vi "MH_WriteTestPTUFileV2.vi"(8 "entrée d'erreur":errorcluster) -> (0 "sortie d'erreur":errorcluster, 3 "refnum Out":refnum<file>)   [LabVIEW 2019]
panel:
  out "Value":u32[](array[numeric])
  out "Records":u32[](array[numeric])
  in  "Path":path
  in  "TagArray":T1(array[cluster])=[{"TagIdent"="File_GUID", "TagIndex"=-1, "TagType"=1073872895, "TagValue"=40, "TagAuxData"="{197B8EE0-02FE-45EA-A6B5-3F8BBDE2D882}\u0000\u0000"}, {"TagIdent"="File_AssuredContent", "TagIndex"=-1, "TagType"=1073872895, "TagValue"=32, "TagAuxData"="MultiHarp: HWSETG SWSETG\u0000\u0000\u0000\u0000\u0000\u0000\u0000\u0000"}, {"TagIdent"="CreatorSW_ContentVersion", "TagIndex"=-1, "TagType"=1073872895, "TagValue"=8, "TagAuxData"="1.0\u0000\u0000\u0000\u0000\u0000"}, {"TagIdent"="CreatorSW_Name", "TagIndex"=-1, "TagType"=1073872895, "TagValue"=16, "TagAuxData"="MultiHarp AcqUI\u0000"}, {"TagIdent"="CreatorSW_Version", "TagIndex"=-1, "TagType"=1073872895, "TagValue"=8, "TagAuxData"="3.0.0.0\u0000"}, {"TagIdent"="File_CreatingTime", "TagIndex"=-1, "TagType"=553648136, "TagValue"=4676398420989345414, "TagAuxData"=""}, {"TagIdent"="File_Comment", "TagIndex"=-1, "TagType"=1073872895, "TagValue"=8, "TagAuxData"="T2 Mode\u0000"}, {"TagIdent"="Measurement_Mode", "TagIndex"=-1, "TagType"=268435464, "TagValue"=2, "TagAuxData"=""}, {"TagIdent"="Measurement_SubMode", "TagIndex"=-1, "TagType"=268435464, "TagValue"=0, "TagAuxData"=""}, {"TagIdent"="TTResult_StopReason", "TagIndex"=-1, "TagType"=268435464, "TagValue"=0, "TagAuxData"=""}, {"TagIdent"="Fast_Load_End", "TagIndex"=-1, "TagType"=-65528, "TagValue"=0, "TagAuxData"=""}, {"TagIdent"="TTResultFormat_TTTRRecType", "TagIndex"=-1, "TagType"=268435464, "TagValue"=66055, "TagAuxData"=""}, {"TagIdent"="TTResultFormat_BitsPerRecord", "TagIndex"=-1, "TagType"=268435464, "TagValue"=32, "TagAuxData"=""}, {"TagIdent"="MeasDesc_BinningFactor", "TagIndex"=-1, "TagType"=268435464, "TagValue"=32, "TagAuxData"=""}, {"TagIdent"="MeasDesc_Offset", "TagIndex"=-1, "TagType"=268435464, "TagValue"=0, "TagAuxData"=""}, {"TagIdent"="MeasDesc_AcquisitionTime", "TagIndex"=-1, "TagType"=268435464, "TagValue"=900000, "TagAuxData"=""}, {"TagIdent"="MeasDesc_StopAt", "TagIndex"=-1, "TagType"=268435464, "TagValue"=4294967295, "TagAuxData"=""}, {"TagIdent"="MeasDesc_StopOnOvfl", "TagIndex"=-1, "TagType"=8, "TagValue"=0, "TagAuxData"=""}, {"TagIdent"="MeasDesc_Restart", "TagIndex"=-1, "TagType"=8, "TagValue"=0, "TagAuxData"=""}, {"TagIdent"="CurSWSetting_DispLog", "TagIndex"=-1, "TagType"=8, "TagValue"=-1, "TagAuxData"=""}, {"TagIdent"="CurSWSetting_DispAxisTimeFrom", "TagIndex"=-1, "TagType"=268435464, "TagValue"=1, "TagAuxData"=""}, {"TagIdent"="CurSWSetting_DispAxisTimeTo", "TagIndex"=-1, "TagType"=268435464, "TagValue"=120, "TagAuxData"=""}, {"TagIdent"="CurSWSetting_DispAxisCountFrom", "TagIndex"=-1, "TagType"=268435464, "TagValue"=1, "TagAuxData"=""}, {"TagIdent"="CurSWSetting_DispAxisCountTo", "TagIndex"=-1, "TagType"=268435464, "TagValue"=10000, "TagAuxData"=""}, {"TagIdent"="CurSWSetting_DispCurves", "TagIndex"=-1, "TagType"=268435464, "TagValue"=16, "TagAuxData"=""}, {"TagIdent"="CurSWSetting_DispCurve_MapTo", "TagIndex"=0, "TagType"=268435464, "TagValue"=0, "TagAuxData"=""}, {"TagIdent"="CurSWSetting_DispCurve_Show", "TagIndex"=0, "TagType"=8, "TagValue"=-1, "TagAuxData"=""}, {"TagIdent"="CurSWSetting_DispCurve_MapTo", "TagIndex"=1, "TagType"=268435464, "TagValue"=1, "TagAuxData"=""}, {"TagIdent"="CurSWSetting_DispCurve_Show", "TagIndex"=1, "TagType"=8, "TagValue"=-1, "TagAuxData"=""}, {"TagIdent"="CurSWSetting_DispCurve_MapTo", "TagIndex"=2, "TagType"=268435464, "TagValue"=2, "TagAuxData"=""}, {"TagIdent"="CurSWSetting_DispCurve_Show", "TagIndex"=2, "TagType"=8, "TagValue"=-1, "TagAuxData"=""}, {"TagIdent"="CurSWSetting_DispCurve_MapTo", "TagIndex"=3, "TagType"=268435464, "TagValue"=3, "TagAuxData"=""}, {"TagIdent"="CurSWSetting_DispCurve_Show", "TagIndex"=3, "TagType"=8, "TagValue"=-1, "TagAuxData"=""}, {"TagIdent"="CurSWSetting_DispCurve_MapTo", "TagIndex"=4, "TagType"=268435464, "TagValue"=4, "TagAuxData"=""}, {"TagIdent"="CurSWSetting_DispCurve_Show", "TagIndex"=4, "TagType"=8, "TagValue"=-1, "TagAuxData"=""}, {"TagIdent"="CurSWSetting_DispCurve_MapTo", "TagIndex"=5, "TagType"=268435464, "TagValue"=5, "TagAuxData"=""}, {"TagIdent"="CurSWSetting_DispCurve_Show", "TagIndex"=5, "TagType"=8, "TagValue"=-1, "TagAuxData"=""}, {"TagIdent"="CurSWSetting_DispCurve_MapTo", "TagIndex"=6, "TagType"=268435464, "TagValue"=6, "TagAuxData"=""}, {"TagIdent"="CurSWSetting_DispCurve_Show", "TagIndex"=6, "TagType"=8, "TagValue"=-1, "TagAuxData"=""}, {"TagIdent"="CurSWSetting_DispCurve_MapTo", "TagIndex"=7, "TagType"=268435464, "TagValue"=7, "TagAuxData"=""}, {"TagIdent"="CurSWSetting_DispCurve_Show", "TagIndex"=7, "TagType"=8, "TagValue"=-1, "TagAuxData"=""}, {"TagIdent"="CurSWSetting_DispCurve_MapTo", "TagIndex"=8, "TagType"=268435464, "TagValue"=8, "TagAuxData"=""}, {"TagIdent"="CurSWSetting_DispCurve_Show", "TagIndex"=8, "TagType"=8, "TagValue"=-1, "TagAuxData"=""}, {"TagIdent"="CurSWSetting_DispCurve_MapTo", "TagIndex"=9, "TagType"=268435464, "TagValue"=9, "TagAuxData"=""}, {"TagIdent"="CurSWSetting_DispCurve_Show", "TagIndex"=9, "TagType"=8, "TagValue"=-1, "TagAuxData"=""}, {"TagIdent"="CurSWSetting_DispCurve_MapTo", "TagIndex"=10, "TagType"=268435464, "TagValue"=10, "TagAuxData"=""}, {"TagIdent"="CurSWSetting_DispCurve_Show", "TagIndex"=10, "TagType"=8, "TagValue"=-1, "TagAuxData"=""}, {"TagIdent"="CurSWSetting_DispCurve_MapTo", "TagIndex"=11, "TagType"=268435464, "TagValue"=11, "TagAuxData"=""}, {"TagIdent"="CurSWSetting_DispCurve_Show", "TagIndex"=11, "TagType"=8, "TagValue"=-1, "TagAuxData"=""}, {"TagIdent"="CurSWSetting_DispCurve_MapTo", "TagIndex"=12, "TagType"=268435464, "TagValue"=12, "TagAuxData"=""}, {"TagIdent"="CurSWSetting_DispCurve_Show", "TagIndex"=12, "TagType"=8, "TagValue"=-1, "TagAuxData"=""}, {"TagIdent"="CurSWSetting_DispCurve_MapTo", "TagIndex"=13, "TagType"=268435464, "TagValue"=13, "TagAuxData"=""}, {"TagIdent"="CurSWSetting_DispCurve_Show", "TagIndex"=13, "TagType"=8, "TagValue"=-1, "TagAuxData"=""}, {"TagIdent"="CurSWSetting_DispCurve_MapTo", "TagIndex"=14, "TagType"=268435464, "TagValue"=14, "TagAuxData"=""}, {"TagIdent"="CurSWSetting_DispCurve_Show", "TagIndex"=14, "TagType"=8, "TagValue"=-1, "TagAuxData"=""}, {"TagIdent"="CurSWSetting_DispCurve_MapTo", "TagIndex"=15, "TagType"=268435464, "TagValue"=15, "TagAuxData"=""}, {"TagIdent"="CurSWSetting_DispCurve_Show", "TagIndex"=15, "TagType"=8, "TagValue"=-1, "TagAuxData"=""}, {"TagIdent"="HW_Type", "TagIndex"=-1, "TagType"=1073872895, "TagValue"=24, "TagAuxData"="MultiHarp 150 4P\u0000\u0000\u0000\u0000\u0000\u0000\u0000\u0000"}, {"TagIdent"="HW_PartNo", "TagIndex"=-1, "TagType"=1073872895, "TagValue"=8, "TagAuxData"="930043\u0000\u0000"}, {"TagIdent"="HW_Version", "TagIndex"=-1, "TagType"=1073872895, "TagValue"=8, "TagAuxData"="1.0\u0000\u0000\u0000\u0000\u0000"}, {"TagIdent"="HW_SerialNo", "TagIndex"=-1, "TagType"=1073872895, "TagValue"=8, "TagAuxData"="1043897\u0000"}, {"TagIdent"="HW_Features", "TagIndex"=-1, "TagType"=285212680, "TagValue"=183, "TagAuxData"=""}, {"TagIdent"="HW_BaseResolution", "TagIndex"=-1, "TagType"=536870920, "TagValue"=4437731733528994965, "TagAuxData"=""}, {"TagIdent"="HW_InpChannels", "TagIndex"=-1, "TagType"=268435464, "TagValue"=4, "TagAuxData"=""}, {"TagIdent"="HW_ExternalRefClock", "TagIndex"=-1, "TagType"=8, "TagValue"=0, "TagAuxData"=""}, {"TagIdent"="HW_ExternalDevices", "TagIndex"=-1, "TagType"=268435464, "TagValue"=0, "TagAuxData"=""}, {"TagIdent"="HWTriggerOut_Period", "TagIndex"=-1, "TagType"=536870920, "TagValue"=4502148214488346441, "TagAuxData"=""}, {"TagIdent"="HWTriggerOut_On", "TagIndex"=-1, "TagType"=8, "TagValue"=0, "TagAuxData"=""}, {"TagIdent"="HW_InputHysteresis", "TagIndex"=-1, "TagType"=8, "TagValue"=0, "TagAuxData"=""}, {"TagIdent"="HWSync_Divider", "TagIndex"=-1, "TagType"=268435464, "TagValue"=1, "TagAuxData"=""}, {"TagIdent"="HWSync_TrgLevel", "TagIndex"=-1, "TagType"=268435464, "TagValue"=-10, "TagAuxData"=""}, {"TagIdent"="HWSync_TrgEdge", "TagIndex"=-1, "TagType"=268435464, "TagValue"=0, "TagAuxData"=""}, {"TagIdent"="HWSync_Offset", "TagIndex"=-1, "TagType"=268435464, "TagValue"=27000, "TagAuxData"=""}, {"TagIdent"="HWSync_TdCode", "TagIndex"=-1, "TagType"=268435464, "TagValue"=0, "TagAuxData"=""}, {"TagIdent"="HWInpChan_TrgLevel", "TagIndex"=0, "TagType"=268435464, "TagValue"=-150, "TagAuxData"=""}, {"TagIdent"="HWInpChan_TrgEdge", "TagIndex"=0, "TagType"=268435464, "TagValue"=0, "TagAuxData"=""}, {"TagIdent"="HWInpChan_Offset", "TagIndex"=0, "TagType"=268435464, "TagValue"=0, "TagAuxData"=""}, {"TagIdent"="HWInpChan_Enabled", "TagIndex"=0, "TagType"=8, "TagValue"=-1, "TagAuxData"=""}, {"TagIdent"="HWInpChan_TdCode", "TagIndex"=0, "TagType"=268435464, "TagValue"=0, "TagAuxData"=""}, {"TagIdent"="HWInpChan_TrgLevel", "TagIndex"=1, "TagType"=268435464, "TagValue"=-150, "TagAuxData"=""}, {"TagIdent"="HWInpChan_TrgEdge", "TagIndex"=1, "TagType"=268435464, "TagValue"=0, "TagAuxData"=""}, {"TagIdent"="HWInpChan_Offset", "TagIndex"=1, "TagType"=268435464, "TagValue"=0, "TagAuxData"=""}, {"TagIdent"="HWInpChan_Enabled", "TagIndex"=1, "TagType"=8, "TagValue"=-1, "TagAuxData"=""}, {"TagIdent"="HWInpChan_TdCode", "TagIndex"=1, "TagType"=268435464, "TagValue"=0, "TagAuxData"=""}, {"TagIdent"="HWInpChan_TrgLevel", "TagIndex"=2, "TagType"=268435464, "TagValue"=-50, "TagAuxData"=""}, {"TagIdent"="HWInpChan_TrgEdge", "TagIndex"=2, "TagType"=268435464, "TagValue"=0, "TagAuxData"=""}, {"TagIdent"="HWInpChan_Offset", "TagIndex"=2, "TagType"=268435464, "TagValue"=0, "TagAuxData"=""}, {"TagIdent"="HWInpChan_Enabled", "TagIndex"=2, "TagType"=8, "TagValue"=-1, "TagAuxData"=""}, {"TagIdent"="HWInpChan_TdCode", "TagIndex"=2, "TagType"=268435464, "TagValue"=0, "TagAuxData"=""}, {"TagIdent"="HWInpChan_TrgLevel", "TagIndex"=3, "TagType"=268435464, "TagValue"=-50, "TagAuxData"=""}, {"TagIdent"="HWInpChan_TrgEdge", "TagIndex"=3, "TagType"=268435464, "TagValue"=0, "TagAuxData"=""}, {"TagIdent"="HWInpChan_Offset", "TagIndex"=3, "TagType"=268435464, "TagValue"=0, "TagAuxData"=""}, {"TagIdent"="HWInpChan_Enabled", "TagIndex"=3, "TagType"=8, "TagValue"=-1, "TagAuxData"=""}, {"TagIdent"="HWInpChan_TdCode", "TagIndex"=3, "TagType"=268435464, "TagValue"=0, "TagAuxData"=""}, {"TagIdent"="MeasDesc_Resolution", "TagIndex"=-1, "TagType"=536870920, "TagValue"=4437731733528994965, "TagAuxData"=""}, {"TagIdent"="HW_Markers", "TagIndex"=-1, "TagType"=268435464, "TagValue"=4, "TagAuxData"=""}, {"TagIdent"="HWMarkers_RisingEdge", "TagIndex"=0, "TagType"=8, "TagValue"=0, "TagAuxData"=""}, {"TagIdent"="HWMarkers_RisingEdge", "TagIndex"=1, "TagType"=8, "TagValue"=0, "TagAuxData"=""}, {"TagIdent"="HWMarkers_RisingEdge", "TagIndex"=2, "TagType"=8, "TagValue"=0, "TagAuxData"=""}, {"TagIdent"="HWMarkers_RisingEdge", "TagIndex"=3, "TagType"=8, "TagValue"=0, "TagAuxData"=""}, {"TagIdent"="HWMarkers_Enabled", "TagIndex"=0, "TagType"=8, "TagValue"=-1, "TagAuxData"=""}, {"TagIdent"="HWMarkers_Enabled", "TagIndex"=1, "TagType"=8, "TagValue"=-1, "TagAuxData"=""}, {"TagIdent"="HWMarkers_Enabled", "TagIndex"=2, "TagType"=8, "TagValue"=-1, "TagAuxData"=""}, {"TagIdent"="HWMarkers_Enabled", "TagIndex"=3, "TagType"=8, "TagValue"=-1, "TagAuxData"=""}, {"TagIdent"="HWMarkers_HoldOff", "TagIndex"=-1, "TagType"=268435464, "TagValue"=0, "TagAuxData"=""}, {"TagIdent"="MeasDesc_GlobalResolution", "TagIndex"=-1, "TagType"=536870920, "TagValue"=4437731733528994965, "TagAuxData"=""}, {"TagIdent"="TTResult_SyncRate", "TagIndex"=-1, "TagType"=268435464, "TagValue"=0, "TagAuxData"=""}, {"TagIdent"="TTResult_InputRate", "TagIndex"=0, "TagType"=268435464, "TagValue"=9126, "TagAuxData"=""}, {"TagIdent"="TTResult_InputRate", "TagIndex"=1, "TagType"=268435464, "TagValue"=8247, "TagAuxData"=""}, {"TagIdent"="TTResult_InputRate", "TagIndex"=2, "TagType"=268435464, "TagValue"=0, "TagAuxData"=""}, {"TagIdent"="TTResult_InputRate", "TagIndex"=3, "TagType"=268435464, "TagValue"=0, "TagAuxData"=""}, {"TagIdent"="TTResult_StopAfter", "TagIndex"=-1, "TagType"=268435464, "TagValue"=130000, "TagAuxData"=""}, {"TagIdent"="TTResult_NumberOfRecords", "TagIndex"=-1, "TagType"=268435464, "TagValue"=130000, "TagAuxData"=""}, {"TagIdent"="TTResult_MDescWarningFlags", "TagIndex"=-1, "TagType"=285212680, "TagValue"=0, "TagAuxData"=""}, {"TagIdent"="Header_End", "TagIndex"=-1, "TagType"=-65528, "TagValue"=0, "TagAuxData"=""}]
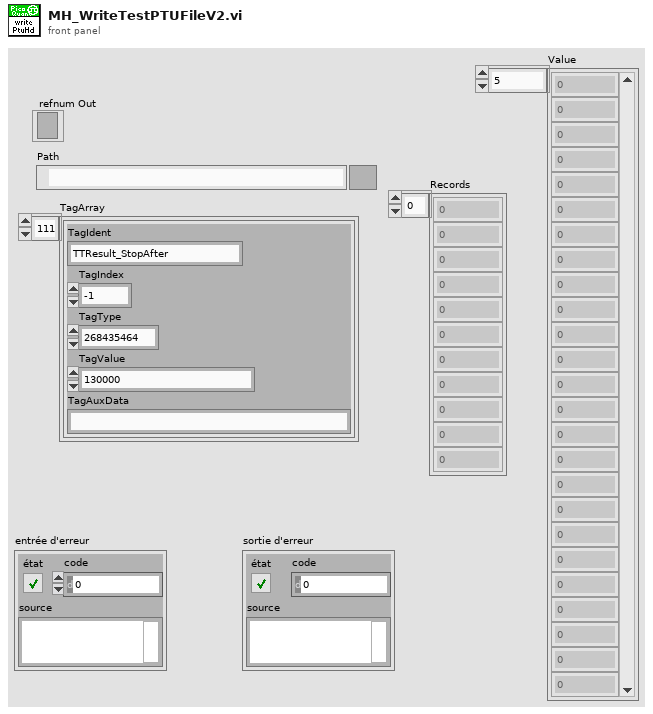
[diagram p1: front panel]
types:
  T1 = cluster{"TagIdent":string, "TagIndex":i32, "TagType":i32, "TagValue":i64, "TagAuxData":string}[]
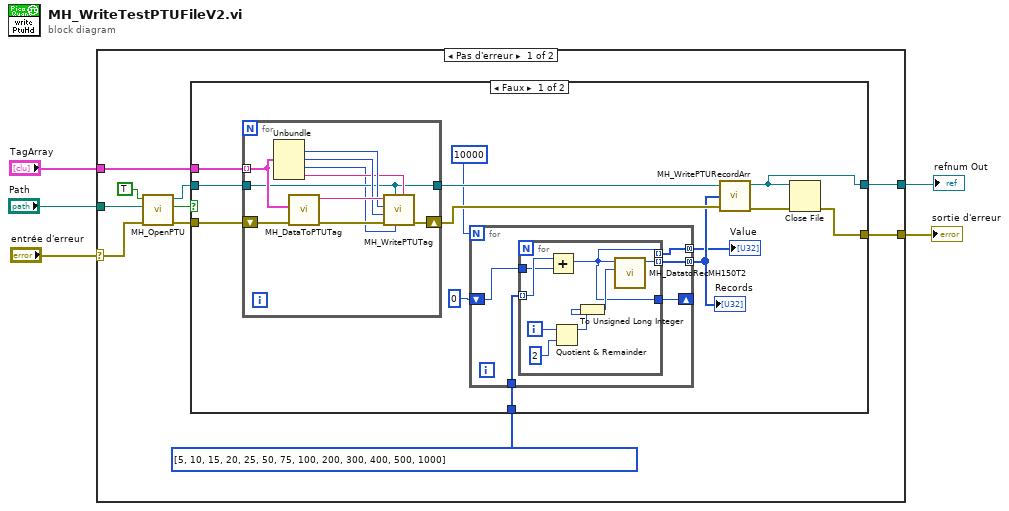
[diagram p0: block diagram]
diagram:
  n1 = case shown="Pas d'erreur" "entrée d'erreur" {
    selector: "entrée d'erreur" -> [w12 w54]
    tunnel: [w15 w54] -> w5
    tunnel: "Path" -> [w10 _]
    tunnel: "TagArray" -> [w8 _]
    tunnel: [w7 _] -> w1
    frame No Error {
      n2 = call <userlib>:"MH_OpenPTU.vi"("ErrorIn"=w12, "chemin sélectionné"=w10, "WriteMode"=TRUE) -> ("ErrorOut"=w13:errorcluster, "Cancelled"=w9:bool, "refnum en sortie"=w14:refnum<file>)  [unwired: 6 in]
      n3 = case shown="Faux" w9 {
        tunnel: w13 -> [w27 w53]
        tunnel: [w25 w53] -> w15
        tunnel: w14 -> [w26 w52]
        tunnel: w8 -> [w28 _]
        tunnel: [w20 w52] -> w7
        tunnel: u32[] [5, 10, 15, 20, 25, 50, 75, 100, 200, 300, 400, 500, 1000] -> [w19 _]
        frame False {
          n4 = for {
            tunnel: w28 -> [w51] mode=indexing
            shift-right: [w44] -> w23
            shift-left: w27 -> [w45]
            tunnel: w26 -> [w43]
            tunnel: [w43] -> w22
            n5 = Unbundle(w51) -> ("TagIndex"=w49:i32, "TagType"=w48:i32, "TagValue"=w42:i64, "TagAuxData"=w47:string)  [unwired: 1 out]
            n6 = call <userlib>:"MH_DataToPTUTag.vi"("error in"=w45, "TagIn"=w51) -> ("error in 2"=w46:errorcluster, "TagIdent Out"=w50:string)  [unwired: 5 in, 3 out]
            n7 = call <userlib>:"MH_WritePTUTag.vi"("TagAuxData"=w47, "TagValue"=w42, "refnum"=w43, "error in"=w46, "TagType"=w48, "TagIndex"=w49, "identifierfull"=w50) -> ("error out"=w44:errorcluster)  [unwired: 3 in]
          }
          n8 = for {
            N: 10000 -> [_]
            tunnel: [w33] -> w21 mode=concatenating
            tunnel: w19 -> [w32]
            shift-right: [w31] -> _
            shift-left: u32 0 ("entier 32 bits non signé") -> [w30]
            tunnel: [w29] -> w16 mode=concatenating
            n9 = for {
              tunnel: [w37] -> w33 mode=indexing
              tunnel: w32 -> [w36] mode=indexing
              tunnel: [w34] -> w31
              tunnel: w30 -> [w35]
              tunnel: [w34] -> w29 mode=indexing
              i -> [w38]
              n10 = Add(x=w36, y=w35) -> (x+y=w34:u32)
              n11 = Quotient & Remainder(x=w38, y=2) -> (x-y*floor(x/y)=w39:i32)  [unwired: 1 out]
              n12 = To Unsigned Long Integer(number=w39) -> (unsigned 32bit integer=w41:u32)
              n13 = call <userlib>:"MH_DatatoRecMH150T2.vi"("channel"=w41, "Time"=w34) -> ("rawbits"=w37:u32)  [unwired: 9 in]
            }
          }
          "Records" <- w21
          "Value" <- w16
          n14 = call <userlib>:"MH_WritePTURecordArr.vi"("refnum"=w22, "TTTR Records"=w21, "error in"=w23) -> ("refnum en sortie"=w20:refnum<file>, "error out"=w24:errorcluster)  [unwired: 6 in]
          n15 = Close File(refnum=w20, error in=w24) -> (error out=w25:errorcluster)  [unwired: 1 out]
        }
        frame True {
        }
      }
    }
    frame Error {
    }
  }
  "sortie d'erreur" <- w5
  "refnum Out" <- w1
